vi "PopulateTreeSumary.vi"(8 "error in":errorcluster, 10 "array":T1[](array[typedef]), 11 "tree ref in":refnum<vi>) -> (0 "error out":errorcluster)   [LabVIEW 2025, in "CEF.lvlib"]
doc: "This VI will populate the tree control with the summary from the nodes. Use this when adding new nodes to treeCopyright 2017 National Instruments Corporation\n\nLicensed under the Apache License, Version 2.0 (the \"License\"); you may not use this file except in compliance with the License. You may obtain a copy of the License at http://www.apache.org/licenses/LICENSE-2.0\nUnless required by applicable law or agreed to in writing, software distributed under the License is distributed on an \"AS IS\" BASIS, WITHOUT WARRANTIES OR CONDITIONS OF ANY KIND, either express or implied. See the License for the specific language governing permissions and limitations under the License."
uses:
  CEF.lvlib
  Node/Summary.ctl
  Node/CEF_Node.lvclass
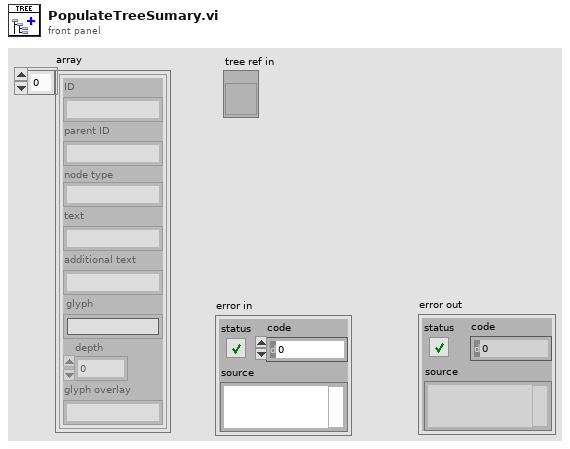
[diagram p1: front panel]
types:
  T1 = typedef "CEF.lvlib/CEF_Node.lvclass/Summary.ctl" = cluster{"ID":string, "parent ID":string, "node type":string, "text":string, "additional text":string, "glyph":string, "depth":i32, "glyph overlay":string}
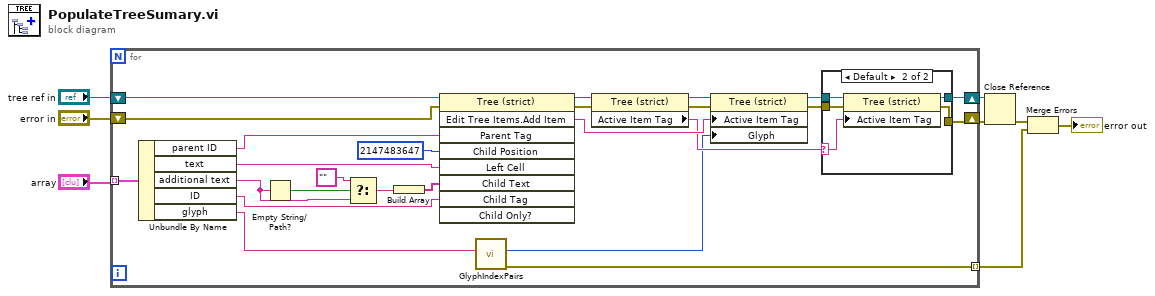
[diagram p0: block diagram]
diagram:
  n1 = for {
    tunnel: "array" -> [w18] mode=indexing
    shift-right: [w14] -> w7
    shift-left: "tree ref in" -> [w17]
    shift-right: [w12] -> w4
    shift-left: "error in" -> [w13]
    tunnel: [w9] -> w3 mode=indexing
    n2 = Unbundle By Name(w18) -> ("parent ID"=w33:string, "text"=w19:string, "additional text"=w11:string, "ID"=w30:string, "glyph"=w16:string)
    n3 = Empty String/Path?(string/path=w11) -> (empty?=w10:bool)
    n4 = Select(t="", s=w10, f=w11) -> (s? t:f=w28:string)
    n5 = Build Array(w28) -> (w31:string[])
    n6 = invoke class="Tree (strict)" method="Edit Tree Items.Add Item"(reference=w17, error in=w13, "Parent Tag"=w33, "Child Position"=2147483647 ("child Position"), "Left Cell"=w19, "Child Text"=w31, "Child Tag"=w30) -> (reference out=w27:refnum<vi>, error out=w26:errorcluster, "Edit Tree Items:Add Item"=w23:string)  [unwired: 2 in, 6 out]
    n7 = call "GlyphIndexPairs.vi"("glyph"=w16) -> ("error out"=w9:errorcluster, "index"=w15:i32)  [unwired: 9 in]
    n8 = property class="Tree (strict)"(reference=w27, error in=w26) -> (reference out=w25:refnum<vi>, error out=w24:errorcluster, "Active Item Tag"=w20:string)
    n9 = property class="Tree (strict)"(reference=w25, error in=w24, "Active Item Tag"=w23, "Glyph"=w15) -> (reference out=w22:refnum<vi>, error out=w21:errorcluster)
    n10 = case shown="Default" w20 {
      selector: w20 -> [_ w38]
      tunnel: w22 -> [w35 w40]
      tunnel: w21 -> [w34 w39]
      tunnel: [w35 w37] -> w14
      tunnel: [w34 w36] -> w12
      frame "" {
      }
      frame Default {
        n11 = property class="Tree (strict)"(reference=w40, error in=w39, "Active Item Tag"=w38) -> (reference out=w37:refnum<vi>, error out=w36:errorcluster)
      }
    }
  }
  n12 = Close Reference(reference=w7, error in (no error)=w4) -> (error out=w2:errorcluster)
  n13 = Merge Errors(w2, w3) -> (→"error out":errorcluster)
